vi "Real to Norm Coordinate.vi"(5 "Zoom":dbl, 7 "FrameSize":dbl, 9 "Y":dbl, 11 "X":dbl) -> (1 "Norm. Y":dbl, 3 "Norm. X":dbl)   [LabVIEW 2017]
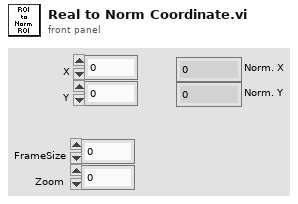
[diagram p1: front panel]
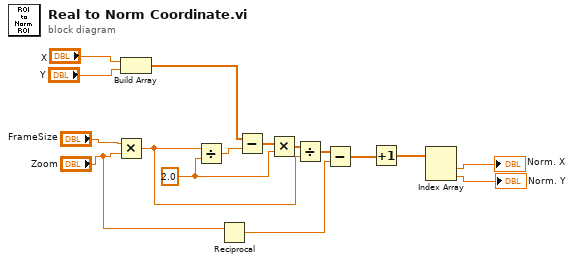
[diagram p0: block diagram]
diagram:
  w14 = 2.0 ("y")
  n1 = Multiply(x="FrameSize", y="Zoom") -> (x*y=w12:dbl)
  n2 = Build Array("X", "Y") -> (w5:dbl[])
  n3 = Divide(x=w12, y=w14) -> (x/y=w13:dbl)
  n4 = Reciprocal(x="Zoom") -> (1/x=w10:dbl)
  n5 = Subtract(x=w5, y=w13) -> (x-y=w15:dbl[])
  n6 = Multiply(x=w15, y=w14) -> (x*y=w16:dbl[])
  n7 = Divide(x=w16, y=w12) -> (x/y=w9:dbl[])
  n8 = Subtract(x=w9, y=w10) -> (x-y=w11:dbl[])
  n9 = Increment(x=w11) -> (x+1=w3:dbl[])
  n10 = Index Array(array=w3) -> (element #1=→"Norm. X":dbl, element #2=→"Norm. Y":dbl)  [unwired: 2 in]
